vi "UDP.Rx.vi"(5 "max size (548)":i32=548, 7 "port":u16=60000, 8 "error in (no error)":errorcluster, 10 "Count Pointer":refnum<class "Memory.Pointer.lvclass">, 11 "Stop Pointer":refnum<class "Memory.Pointer.lvclass">) -> (0 "error out":errorcluster)   [LabVIEW 2017]
uses:
  <vilib>/National Instruments/Memory Manager/Classes/Pointer/Memory.Pointer.lvclass
  <vilib>/National Instruments/Memory Manager/Classes/Pointer/Memory.Pointer.lvclass/Memory.Pointer.ctl
  <vilib>/National Instruments/Memory Manager/Classes/Pointer/Memory.Pointer.Read.0D.Bool.vi
  <vilib>/National Instruments/Memory Manager/Classes/Pointer/Memory.Pointer.Write.0D.I32.vi
  <vilib>/National Instruments/Memory Manager/Classes/Pointer/Memory.Pointer.Write.0D.Bool.vi
  <vilib>/National Instruments/Memory Manager/Classes/Pointer/Memory.Pointer.Read.No Check.0D.Bool.vi
  <vilib>/National Instruments/Memory Manager/Classes/Pointer/Memory.Pointer.Parameter Check.Null Pointer.vi
  <vilib>/National Instruments/Memory Manager/Classes/Pointer/Memory.Pointer.Parameter Check.Subset.vi
  <vilib>/National Instruments/Memory Manager/Classes/Pointer/Memory.Pointer.Write.No Check.0D.I32.vi
  <vilib>/National Instruments/Memory Manager/Classes/Pointer/Memory.Pointer.Write.No Check.0D.Bool.vi
  <vilib>/National Instruments/Memory Manager/Classes/Pointer/Memory.Pointer.Get Address.vi
  <vilib>/National Instruments/Memory Manager/Classes/Pointer/Memory.Pointer.Errors.vi
  <vilib>/National Instruments/Memory Manager/Classes/Pointer/Memory.Pointer.Errors.Null Pointer.vi
  <vilib>/National Instruments/Memory Manager/Classes/Pointer/Memory.Pointer.Errors.Out of Bounds.vi
  <vilib>/National Instruments/Memory Manager/Classes/Pointer/Memory.Pointer.Get Size.vi
  <vilib>/National Instruments/Memory Manager/Classes/Pointer/Memory.Pointer.Errors.Create Error.vi
  <vilib>/NI/Static Error Handling/VIs/Static Error Handling.Source Buffer.Write.String.vi
  <vilib>/National Instruments/Memory Manager/Classes/Pointer/Memory.Pointer.Errors.Write Pointer Size.vi
  <vilib>/NI/Static Error Handling/VIs/Static Error Handling.Source Buffer.Write.Numeric.Scalar.Base10.vi
  <vilib>/NI/Static Error Handling/VIs/Static Error Handling.Source Buffer.Write.Numeric.Scalar.Base10 (U64).vi
  <vilib>/NI/Static Error Handling/VIs/Static Error Handling.Error Cluster Constant.vi
  <vilib>/NI/Static Error Handling/VIs/Static Error Handling.Error Cluster Constant (512B).vi
  <vilib>/NI/Static Error Handling/VIs/Static Error Handling.Parameters.Status.Set.vi
  <vilib>/NI/Static Error Handling/VIs/Static Error Handling.Parameters.Code.Set.vi
  <vilib>/NI/Static Error Handling/VIs/Static Error Handling.Parameters.VI Source.Set.vi
  <vilib>/National Instruments/Memory Manager/Constants/Memory.Constants.vi
  <vilib>/National Instruments/Memory Manager/Constants/Memory.Constants.Library Name.vi
  <vilib>/National Instruments/Memory Manager/Classes/Pointer/Memory.Pointer.Errors.Get Info.vi
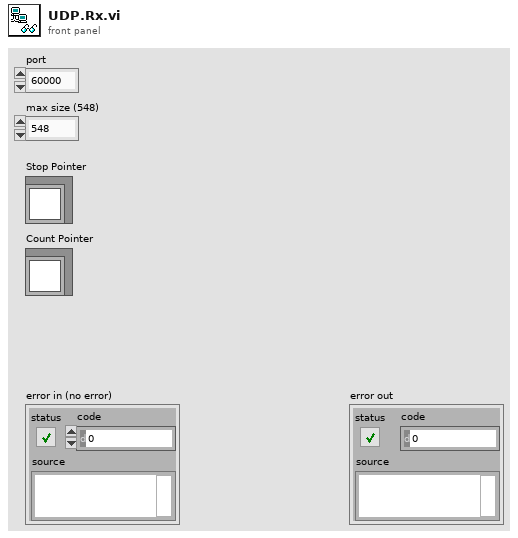
[diagram p1: front panel]
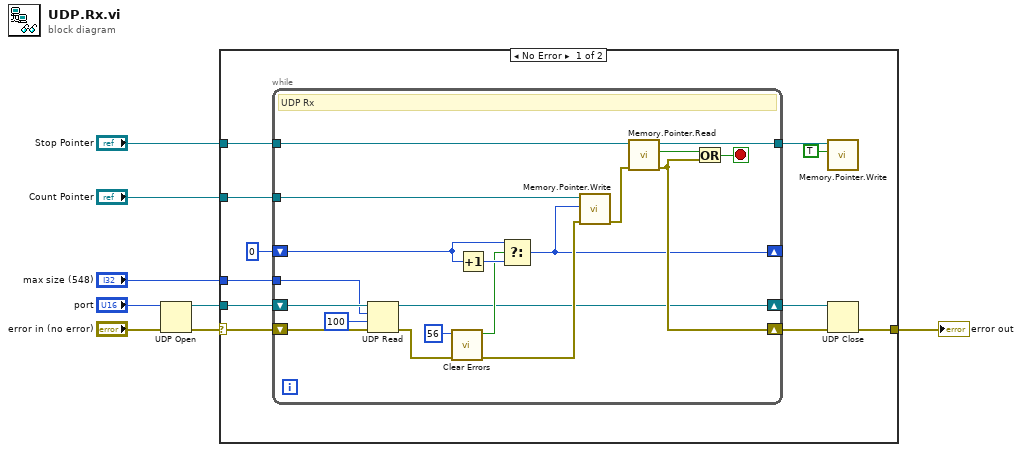
[diagram p0: block diagram]
diagram:
  n1 = UDP Open(8:"error in (no error)", 11:"port") -> (port=w8:refnum<k16>, 0:w2:errorcluster)  [unwired: 3 in, 1 out]
  n2 = case shown="No Error" w2 {
    selector: w2 -> [w12 w39]
    tunnel: w8 -> [w19 _]
    tunnel: "max size (548)" -> [w18 _]
    tunnel: "Stop Pointer" -> [w16 _]
    tunnel: "Count Pointer" -> [w15 _]
    tunnel: [w9 w39] -> w1
    frame No Error {
      n3 = while {
        shift-right: [w23] -> w11
        shift-left: w12 -> [w37]
        shift-right: [w21] -> w10
        shift-left: w19 -> [w38]
        tunnel: w16 -> [w29]
        tunnel: w18 -> [w35]
        shift-right: [w22] -> _
        shift-left: 0 -> [w31]
        tunnel: w15 -> [w27]
        tunnel: [w20] -> w14
        stop <- w36 stop-if-true
        # "UDP Rx"
        n4 = UDP Read(connection ID=w38, max size (548)=w35, timeout ms (25000)=100, 8:w37) -> (error out=w32:errorcluster, 3:w21:refnum<k16>)  [unwired: 3 out]
        n5 = call <vilib>:"Clear Errors.vi"("error in (no error)"=w32, "specific error code to clear (0: all)"=56) -> ("error out"=w25:errorcluster, "specific error cleared?"=w28:bool)  [unwired: 4 in]
        n6 = Increment(x=w31) -> (x+1=w30:i32)
        n7 = Select(t=w31, s=w28, f=w30) -> (s? t:f=w22:i32)
        n8 = call-poly <vilib>:"Memory.Pointer.Write.vi"("error in (no error)"=w25, "value"=w22, "Pointer in"=w27) -> ("error out"=w24:errorcluster)  [unwired: 5 in, 3 out]
        n9 = call-poly <vilib>:"Memory.Pointer.Read.vi"("error in (no error)"=w24, "Pointer in"=w29) -> ("error out"=w23:errorcluster, "value out"=w26:bool, "Pointer out"=w20:refnum<class "Memory.Pointer.lvclass">)  [unwired: 6 in, 1 out]
        n10 = Or(x=w26, y=w23) -> (x .or. y?=w36:bool)
      }
      n11 = call-poly <vilib>:"Memory.Pointer.Write.vi"("value"=TRUE, "Pointer in"=w14) -> ()  [unwired: 6 in, 4 out]
      n12 = UDP Close(connection ID=w10, 8:w11) -> (error out=w9:errorcluster)  [unwired: 1 out]
    }
    frame Error {
    }
  }
  "error out" <- w1
